vi "GlobalCancel-StatusDisplay.vi"() -> ()   [LabVIEW 2024]
uses:
  Globals and TypeDefs/Type Definitions.llb/3 way Status.ctl
  Globals and TypeDefs/Type Definitions.llb/McPherson Status.ctt
  Globals and TypeDefs/gStatus.vi
  Globals and TypeDefs/gHField.vi
  Globals and TypeDefs/gGeneral.vi
  Globals and TypeDefs/gSpectrometer.vi
panel:
  in  "quit":bool
  in  "Tab Control":enum32{"1", "G"}(tab)
  in  "Close Global":bool
  in  "Open Global":bool
  out "Spectrometer Pos":T2
  out "Saving":T3 items=["N.A.", "OK", "Busy", "Done"]
  out "Plotting":T3 items=["N.A.", "OK", "Busy", "Done"]
  out "Buffer":T3 items=["N.A.", "OK", "Busy", "Done"]
  in  "Stop-All":bool
  in  "Resume":bool
  in  "Cancel":bool
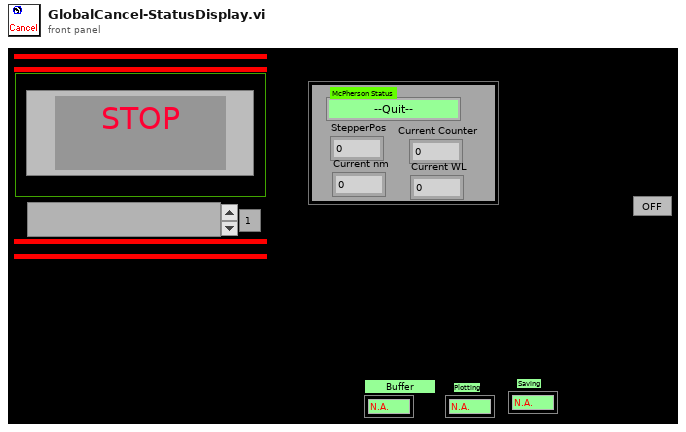
[diagram p1: front panel]
types:
  T1 = typedef "McPherson Status.ctt" = enum8{"--Quit--", "Error", "Initialization", "Standby", "Start Slew", "-Slew", "+Slew", "Slew Done", "Start Scan", "-Slew to Start", "+Slew to Start", "Scanning", "Scan Done", "Scan Pause", "Slew Pause", "Cancel", "Update Z0", "Sleep"}
  T2 = cluster{"StepperPos":i32, "Current nm":dbl, "Current Counter":dbl, "Current WL":dbl, "McPherson Status":T1}
  T3 = typedef "3 way Status.ctl" = u8
  T4 = cluster{"Field [T]":dbl, "Status":cluster{bool, bool, "Ramp Status":u16, bool}}
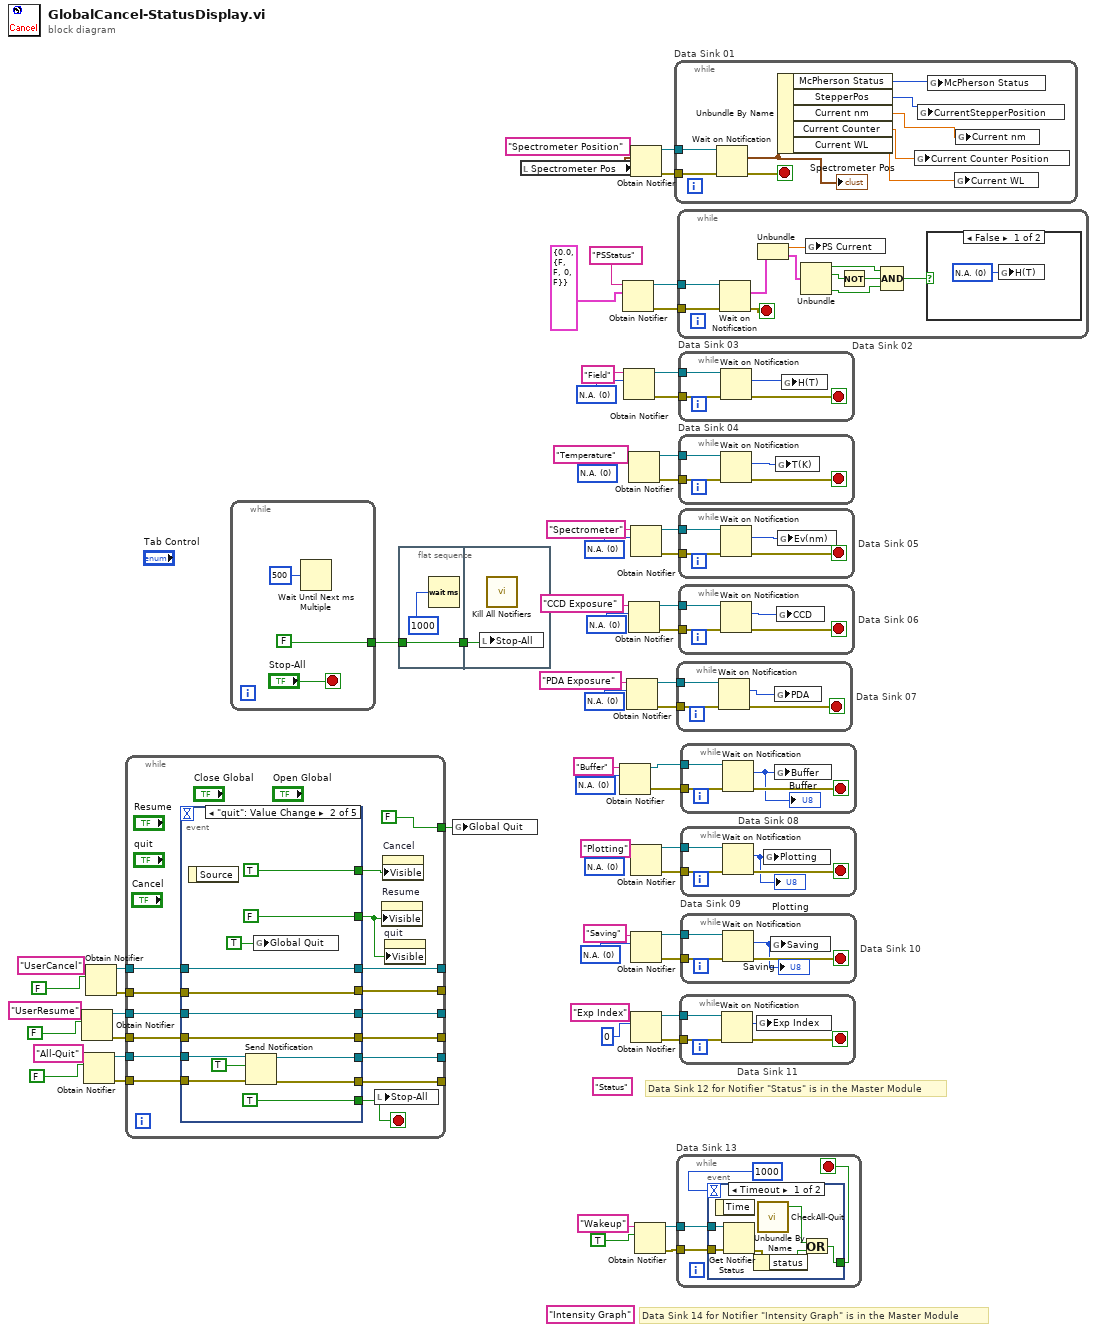
[diagram p0: block diagram]
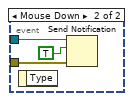
[diagram p2: hidden frame]
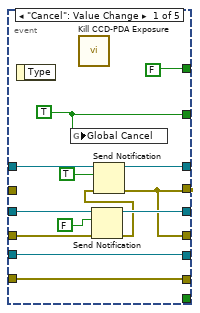
[diagram p4: hidden frame]
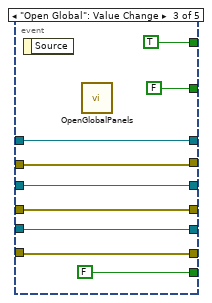
[diagram p5: hidden frame]
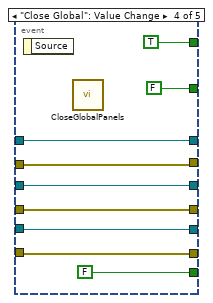
[diagram p6: hidden frame]
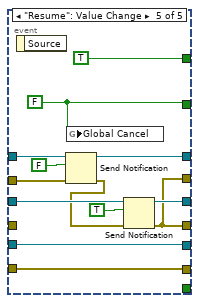
[diagram p7: hidden frame]
diagram:
  (unwired) "Intensity Graph" ("name (unnamed)")
  w18 = T3 0 items=["N.A.", "OK", "Busy", "Done"] ("Saving")
  (unwired) "Status" ("name (unnamed)")
  w50 = T3 0 items=["N.A.", "OK", "Busy", "Done"] ("Saving")
  w52 = T3 0 items=["N.A.", "OK", "Busy", "Done"] ("Saving")
  w54 = T3 0 items=["N.A.", "OK", "Busy", "Done"] ("Saving")
  w55 = T3 0 items=["N.A.", "OK", "Busy", "Done"] ("Saving")
  w57 = T3 0 items=["N.A.", "OK", "Busy", "Done"] ("Saving")
  w59 = T3 0 items=["N.A.", "OK", "Busy", "Done"] ("Saving")
  w61 = T3 0 items=["N.A.", "OK", "Busy", "Done"] ("Saving")
  # "Data Sink 14 for Notifier \"Intensity Graph\" is in the Master Module"
  # "Data Sink 12 for Notifier \"Status\" is in the Master Module"
  n1 = Obtain Notifier(name (unnamed)="UserResume", notification data type=FALSE) -> (notifier out=w12:refnum<notifier>, error out=w11:errorcluster)  [unwired: 2 in, 1 out]
  n2 = Obtain Notifier(name (unnamed)="All-Quit", notification data type=FALSE) -> (notifier out=w24:refnum<notifier>, error out=w23:errorcluster)  [unwired: 2 in, 1 out]
  n3 = Obtain Notifier(name (unnamed)="UserCancel", notification data type=FALSE) -> (notifier out=w28:refnum<notifier>, error out=w27:errorcluster)  [unwired: 2 in, 1 out]
  n4 = while {
    tunnel: w28 -> [w76]
    tunnel: w27 -> [w75]
    tunnel: [w74] -> _
    tunnel: w24 -> [w73]
    tunnel: w23 -> [w72]
    tunnel: [w71] -> _
    tunnel: [w70] -> _
    tunnel: w12 -> [w69]
    tunnel: [w68] -> _
    tunnel: w11 -> [w67]
    tunnel: [w66] -> _
    tunnel: [w65] -> _
    tunnel: [FALSE] -> w1
    stop <- w77 stop-if-true
    n5 = event shown="[1] \"quit\": Value Change" {
      selector: _ -> [_ _ _ _ _]
      dyn-events: _ -> [_ _ _ _ _]
      timeout: _ -> [_ _ _ _ _]
      tunnel: [FALSE TRUE TRUE TRUE TRUE] -> w79
      tunnel: [w92 FALSE FALSE FALSE w135] -> w78
      tunnel: [_ TRUE FALSE FALSE _] -> w77
      tunnel: w76 -> [w90 w102 w111 w120 w128]
      tunnel: w75 -> [_ w101 w110 w119 w127]
      tunnel: [w80 w101 w110 w119 w124] -> w65
      tunnel: [w88 w102 w111 w120 w126] -> w74
      tunnel: w73 -> [w87 w100 w107 w116 w134]
      tunnel: w72 -> [w86 w99 w106 w115 w133]
      tunnel: [w87 w98 w107 w116 w134] -> w71
      tunnel: [w86 w97 w106 w115 w133] -> w70
      tunnel: [w84 w95 w109 w118 w130] -> w68
      tunnel: w69 -> [w83 w95 w109 w118 w131]
      tunnel: w67 -> [w82 w94 w108 w117 _]
      tunnel: [w80 w94 w108 w117 w124] -> w66
      event "Cancel": Value Change {
        w92 = TRUE
        n6 = event-data() -> ()  [unwired: 1 in, 1 out]
        n7 = global write "gGeneral.vi" "Global Cancel"(w92) -> ()
        n8 = call "Kill CCD-PDA Exposure.vi"() -> ()  [unwired: 1 in]
        n9 = Send Notification(notification=FALSE, notifier=w83, error in (no error)=w82) -> (notifier out=w84:refnum<notifier>, error out=w81:errorcluster)
        n10 = Send Notification(notification=TRUE, notifier=w90, error in (no error)=w81) -> (notifier out=w88:refnum<notifier>, error out=w80:errorcluster)
      }
      event "quit": Value Change {
        n11 = event-data() -> ()  [unwired: 1 in, 1 out]
        n12 = Send Notification(notification=TRUE, notifier=w100, error in (no error)=w99) -> (notifier out=w98:refnum<notifier>, error out=w97:errorcluster)
        n13 = global write "gGeneral.vi" "Global Quit"(TRUE ("Global Quit")) -> ()
      }
      event "Open Global": Value Change {
        n14 = event-data() -> ()  [unwired: 1 in, 1 out]
        n15 = call "OpenGlobalPanels.vi"() -> ()  [unwired: 1 in]
      }
      event "Close Global": Value Change {
        n16 = event-data() -> ()  [unwired: 1 in, 1 out]
        n17 = call "CloseGlobalPanels.vi"() -> ()  [unwired: 1 in]
      }
      event "Resume": Value Change {
        w135 = FALSE
        n18 = event-data() -> ()  [unwired: 1 in, 1 out]
        n19 = Send Notification(notification=FALSE, notifier=w128, error in (no error)=w127) -> (notifier out=w126:refnum<notifier>, error out=w125:errorcluster)
        n20 = global write "gGeneral.vi" "Global Cancel"(w135) -> ()
        n21 = Send Notification(notification=TRUE, notifier=w131, error in (no error)=w125) -> (notifier out=w130:refnum<notifier>, error out=w124:errorcluster)
      }
    }
    n22 = local write "Stop-All"(w77) -> ()
    n23 = property on="Resume" class="Bool"("Visible"=w78) -> ()  [unwired: 2 in, 2 out]
    n24 = property on="Cancel" class="Bool"("Visible"=w79) -> ()  [unwired: 2 in, 2 out]
    n25 = property on="quit" class="Bool"("Visible"=w78) -> ()  [unwired: 2 in, 2 out]
  }
  n26 = while {
    tunnel: [FALSE] -> w63
    stop <- "Stop-All" stop-if-true
    n27 = Wait Until Next ms Multiple(millisecond multiple=u32 500) -> ()  [unwired: 1 out]
  }
  n28 = flat-sequence {
    tunnel: w63 -> [w141]
    tunnel: [w141] -> w2
    tunnel: w2 -> [w142]
    frame #0 {
      n29 = Wait (ms)(milliseconds to wait=u32 1000) -> ()  [unwired: 1 out]
    }
    frame #1 {
      n30 = local write "Stop-All"(w142) -> ()
      n31 = call "Kill All Notifiers.vi"() -> ()  [unwired: 1 in]
    }
  }
  n32 = global write "gGeneral.vi" "Global Quit"(w1) -> ()
  n33 = local read "Spectrometer Pos"() -> (w7:T2)
  n34 = Obtain Notifier(name (unnamed)="Buffer", notification data type=w52) -> (notifier out=w38:refnum<notifier>, error out=w37:errorcluster)  [unwired: 2 in, 1 out]
  n35 = Obtain Notifier(name (unnamed)="PSStatus", notification data type=T4 {"Field [T]"=0.0, "Status"={FALSE, FALSE, "Ramp Status"=0, FALSE}} ("output cluster")) -> (notifier out=w21:refnum<notifier>, error out=w20:errorcluster)  [unwired: 2 in, 1 out]
  n36 = Obtain Notifier(name (unnamed)="Field", notification data type=w59) -> (notifier out=w44:refnum<notifier>, error out=w43:errorcluster)  [unwired: 2 in, 1 out]
  n37 = Obtain Notifier(name (unnamed)="PDA Exposure", notification data type=w18) -> (notifier out=w15:refnum<notifier>, error out=w16:errorcluster)  [unwired: 2 in, 1 out]
  n38 = Obtain Notifier(name (unnamed)="Temperature", notification data type=w57) -> (notifier out=w32:refnum<notifier>, error out=w31:errorcluster)  [unwired: 2 in, 1 out]
  n39 = Obtain Notifier(name (unnamed)="CCD Exposure", notification data type=w54) -> (notifier out=w35:refnum<notifier>, error out=w36:errorcluster)  [unwired: 2 in, 1 out]
  n40 = Obtain Notifier(name (unnamed)="Spectrometer Position", notification data type=w7) -> (notifier out=w9:refnum<notifier>, error out=w8:errorcluster)  [unwired: 2 in, 1 out]
  n41 = Obtain Notifier(name (unnamed)="Spectrometer", notification data type=w55) -> (notifier out=w34:refnum<notifier>, error out=w33:errorcluster)  [unwired: 2 in, 1 out]
  n42 = Obtain Notifier(name (unnamed)="Plotting", notification data type=w50) -> (notifier out=w40:refnum<notifier>, error out=w39:errorcluster)  [unwired: 2 in, 1 out]
  n43 = Obtain Notifier(name (unnamed)="Saving", notification data type=w61) -> (notifier out=w42:refnum<notifier>, error out=w41:errorcluster)  [unwired: 2 in, 1 out]
  n44 = Obtain Notifier(name (unnamed)="Exp Index", notification data type=u32 0 ("Exp Index")) -> (notifier out=w46:refnum<notifier>, error out=w45:errorcluster)  [unwired: 2 in, 1 out]
  n45 = Obtain Notifier(name (unnamed)="Wakeup", notification data type=TRUE) -> (notifier out=w4:refnum<notifier>, error out=w5:errorcluster)  [unwired: 2 in, 1 out]
  n46 = while "Data Sink 01" {
    tunnel: w9 -> [w149]
    tunnel: w8 -> [w151]
    stop <- w150 stop-if-true
    n47 = Wait on Notification(notifier=w149, error in (no error)=w151) -> (notification=w144:T2, error out=w150:errorcluster)  [unwired: 2 in, 2 out]
    "Spectrometer Pos" <- w144
    n48 = Unbundle By Name(w144) -> ("McPherson Status"=w143:T1, "StepperPos"=w148:i32, "Current nm"=w147:dbl, "Current Counter"=w146:dbl, "Current WL"=w145:dbl)
    n49 = global write "gSpectrometer.vi" "Current Counter Position"(w146) -> ()
    n50 = global write "gSpectrometer.vi" "CurrentStepperPosition"(w148) -> ()
    n51 = global write "gSpectrometer.vi" "McPherson Status"(w143) -> ()
    n52 = global write "gSpectrometer.vi" "Current WL"(w145) -> ()
    n53 = global write "gSpectrometer.vi" "Current nm"(w147) -> ()
  }
  n54 = while "Data Sink 07" {
    tunnel: w15 -> [w153]
    tunnel: w16 -> [w155]
    stop <- w154 stop-if-true
    n55 = Wait on Notification(notifier=w153, error in (no error)=w155) -> (notification=w152:T3, error out=w154:errorcluster)  [unwired: 2 in, 2 out]
    n56 = global write "gStatus.vi" "PDA"(w152) -> ()
  }
  n57 = while "Data Sink 13" {
    tunnel: w4 -> [w157]
    tunnel: w5 -> [w158]
    stop <- w156 stop-if-true
    n58 = event shown="[0] Timeout" {
      selector: _ -> [_ _]
      dyn-events: _ -> [_ _]
      timeout: 1000 -> [_ _]
      tunnel: w158 -> [w161 w167]
      tunnel: w157 -> [w162 w168]
      tunnel: [w163 _] -> w156
      event Timeout {
        n59 = event-data() -> ()  [unwired: 1 in, 1 out]
        n60 = Get Notifier Status(notifier=w162, error in (no error)=w161) -> (error out=w160:errorcluster)  [unwired: 4 out]
        n61 = Unbundle By Name(w160) -> ("status"=w165:bool)
        n62 = call "CheckAll-Quit.vi"() -> ("All-Quit"=w164:bool)  [unwired: 3 in]
        n63 = Or(x=w164, y=w165) -> (x .or. y?=w163:bool)
      }
      event Mouse Down {
        n64 = event-data() -> ()  [unwired: 1 in, 1 out]
        n65 = Send Notification(notification=TRUE, notifier=w168, error in (no error)=w167) -> ()  [unwired: 2 out]
      }
    }
  }
  n66 = while "Data Sink 02" {
    tunnel: w21 -> [w177]
    tunnel: w20 -> [w179]
    stop <- w178 stop-if-true
    n67 = Wait on Notification(notifier=w177, error in (no error)=w179) -> (notification=w176:T4, error out=w178:errorcluster)  [unwired: 2 in, 2 out]
    n68 = Unbundle(w176) -> ("Field [T]"=w175:dbl, "Status"=w172:cluster{bool, bool, "Ramp Status":u16, bool})
    n69 = Unbundle(w172) -> (w174:bool, w171:bool, w169:bool)  [unwired: 1 out]
    n70 = global write "gHField.vi" "PS Current"(w175) -> ()
    n71 = Not(x=w171) -> (.not. x?=w170:bool)
    n72 = Compound Arithmetic op=AND(w174, w170, w169) -> (w173:bool)
    n73 = case shown="False" w173 {
      frame False {
        w180 = T3 0 items=["N.A.", "OK", "Busy", "Done"] ("H(T)")
        n74 = global write "gStatus.vi" "H(T)"(w180) -> ()
      }
      frame True {
      }
    }
  }
  n75 = while "Data Sink 03" {
    tunnel: w44 -> [w182]
    tunnel: w43 -> [w184]
    stop <- w183 stop-if-true
    n76 = Wait on Notification(notifier=w182, error in (no error)=w184) -> (notification=w181:T3, error out=w183:errorcluster)  [unwired: 2 in, 2 out]
    n77 = global write "gStatus.vi" "H(T)"(w181) -> ()
  }
  n78 = while "Data Sink 04" {
    tunnel: w32 -> [w186]
    tunnel: w31 -> [w188]
    stop <- w187 stop-if-true
    n79 = Wait on Notification(notifier=w186, error in (no error)=w188) -> (notification=w185:T3, error out=w187:errorcluster)  [unwired: 2 in, 2 out]
    n80 = global write "gStatus.vi" "T(K)"(w185) -> ()
  }
  n81 = while "Data Sink 05" {
    tunnel: w34 -> [w190]
    tunnel: w33 -> [w192]
    stop <- w191 stop-if-true
    n82 = Wait on Notification(notifier=w190, error in (no error)=w192) -> (notification=w189:T3, error out=w191:errorcluster)  [unwired: 2 in, 2 out]
    n83 = global write "gStatus.vi" "Ev(nm)"(w189) -> ()
  }
  n84 = while "Data Sink 06" {
    tunnel: w35 -> [w194]
    tunnel: w36 -> [w196]
    stop <- w195 stop-if-true
    n85 = Wait on Notification(notifier=w194, error in (no error)=w196) -> (notification=w193:T3, error out=w195:errorcluster)  [unwired: 2 in, 2 out]
    n86 = global write "gStatus.vi" "CCD"(w193) -> ()
  }
  n87 = while "Data Sink 11" {
    tunnel: w46 -> [w198]
    tunnel: w45 -> [w200]
    stop <- w199 stop-if-true
    n88 = Wait on Notification(notifier=w198, error in (no error)=w200) -> (notification=w197:u32, error out=w199:errorcluster)  [unwired: 2 in, 2 out]
    n89 = global write "gStatus.vi" "Exp Index"(w197) -> ()
  }
  n90 = while "Data Sink 08" {
    tunnel: w38 -> [w202]
    tunnel: w37 -> [w204]
    stop <- w203 stop-if-true
    n91 = Wait on Notification(notifier=w202, error in (no error)=w204) -> (notification=w201:T3, error out=w203:errorcluster)  [unwired: 2 in, 2 out]
    "Buffer" <- w201
    n92 = global write "gStatus.vi" "Buffer"(w201) -> ()
  }
  n93 = while "Data Sink 09" {
    tunnel: w40 -> [w206]
    tunnel: w39 -> [w208]
    stop <- w207 stop-if-true
    n94 = Wait on Notification(notifier=w206, error in (no error)=w208) -> (notification=w205:T3, error out=w207:errorcluster)  [unwired: 2 in, 2 out]
    "Plotting" <- w205
    n95 = global write "gStatus.vi" "Plotting"(w205) -> ()
  }
  n96 = while "Data Sink 10" {
    tunnel: w42 -> [w210]
    tunnel: w41 -> [w212]
    stop <- w211 stop-if-true
    n97 = Wait on Notification(notifier=w210, error in (no error)=w212) -> (notification=w209:T3, error out=w211:errorcluster)  [unwired: 2 in, 2 out]
    "Saving" <- w209
    n98 = global write "gStatus.vi" "Saving"(w209) -> ()
  }
